vi "Pack Waveforms.vi"(11 "waveforms":waveform(dbl)[](array[waveform])) -> (3 "packed waveforms":dbl[][](array[numeric]))   [LabVIEW 2024, in "Dynamic Signal Acquisition (Interactive).lvlib"]
uses:
  Dynamic Signal Acquisition (Interactive).lvlib
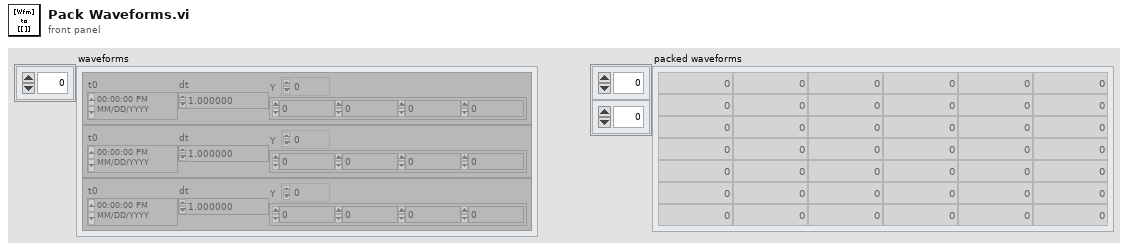
[diagram p1: front panel]
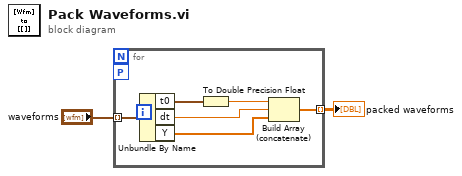
[diagram p0: block diagram]
diagram:
  n1 = for {
    workers-P: _ -> [_]
    tunnel: "waveforms" -> [w7] mode=indexing
    tunnel: [w3] -> w1 mode=indexing
    n2 = Unbundle By Name(w7) -> ("t0"=w8:timestamp, "dt"=w5:dbl, "Y"=w4:dbl[])
    n3 = To Double Precision Float(number=w8) -> (double precision float=w6:dbl)
    n4 = Build Array (concatenate)(w6, w5, w4) -> (w3:dbl[])
  }
  "packed waveforms" <- w1
